vi "AlliGator Read HDF5 FLI Dataset Series Timestamps.vi"(8 "error in (no error)":errorcluster, 11 "File Paths":path[](array[path])) -> (0 "error out":errorcluster, 2 "Timestamps":dbl[](array[numeric]), 3 "File Paths (dup)":path[](array[path]))   [LabVIEW 2021, in "AlliGator HDF5.lvlib"]
doc: "Loads HDF5 FLI dataset gate images timestamps"
uses:
  AlliGator HDF5.lvlib
  <vilib>/addons/h5labview2/base/lib_path.vi
  <vilib>/addons/h5labview2/base/H5Equery.vi
  <vilib>/addons/h5labview2/base/hid_t.ctl
  <vilib>/addons/h5labview2/dataset/H5Dread.llb/H5Dread.xnode
  <vilib>/addons/h5labview2/file/H5F.lvlib
  <vilib>/addons/h5labview2/group/H5G.lvlib
  Error/Error.lvlib
panel:
  # "see the AlliGator License on the block diagram (Ctrl+E or Window:Show Block Diagram)"
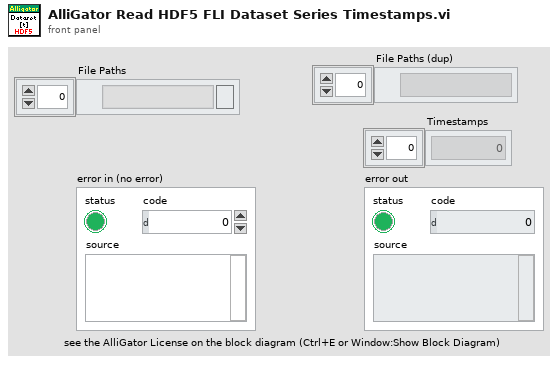
[diagram p1: front panel]
types:
  T1 = typedef "hid_t.ctl" = i64
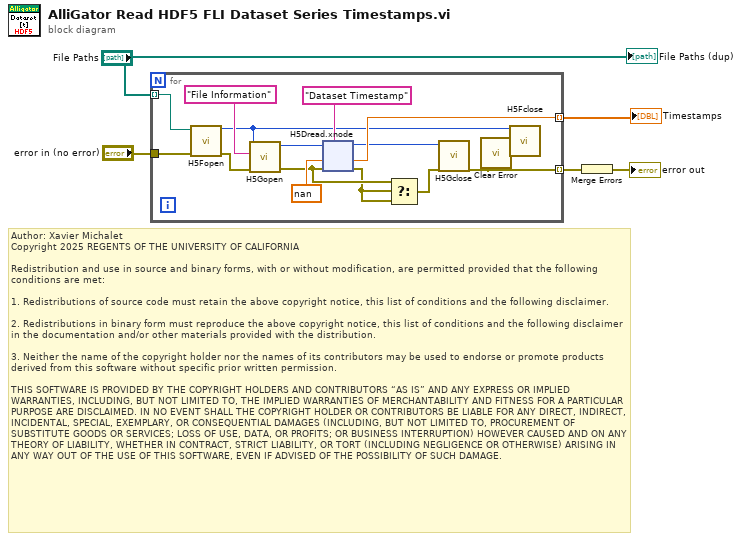
[diagram p0: block diagram]
diagram:
  # "Author: Xavier Michalet\nCopyright 2025 REGENTS OF THE UNIVERSITY OF CALIFORNIA\n\nRedistribution and use in source and binary forms, with or without modification, are permitted provided that the following conditions are met:\n\n1. Redistributions of source code must retain the above copyright notice, this list of conditions and the following disclaimer.\n\n2. Redistributions in binary form must reproduce the above copyright notice, this list of conditions and the following disclaimer in the documentation and/or other materials provided with the distribution.\n\n3. Neither the name of the copyright holder nor the names of its contributors may be used to endorse or promote products derived from this software without specific prior written permission.\n\nTHIS SOFTWARE IS PROVIDED BY THE COPYRIGHT HOLDERS AND CONTRIBUTORS “AS IS” AND ANY EXPRESS OR IMPLIED WARRANTIES, INCLUDING, BUT NOT LIMITED TO, THE IMPLIED WARRANTIES OF MERCHANTABILITY AND FITNESS FOR A PARTICULAR PURPOSE ARE DISCLAIMED. IN NO EVENT SHALL THE COPYRIGHT HOLDER OR CONTRIBUTORS BE LIABLE FOR ANY DIRECT, INDIRECT, INCIDENTAL, SPECIAL, EXEMPLARY, OR CONSEQUENTIAL DAMAGES (INCLUDING, BUT NOT LIMITED TO, PROCUREMENT OF SUBSTITUTE GOODS OR SERVICES; LOSS OF USE, DATA, OR PROFITS; OR BUSINESS INTERRUPTION) HOWEVER CAUSED AND ON ANY THEORY OF LIABILITY, WHETHER IN CONTRACT, STRICT LIABILITY, OR TORT (INCLUDING NEGLIGENCE OR OTHERWISE) ARISING IN ANY WAY OUT OF THE USE OF THIS SOFTWARE, EVEN IF ADVISED OF THE POSSIBILITY OF SUCH DAMAGE."
  n1 = for {
    tunnel: "File Paths" -> [w20] mode=indexing
    tunnel: "error in (no error)" -> [w19]
    tunnel: [w13] -> w3 mode=indexing
    tunnel: [w10] -> w2 mode=indexing
    n2 = call <vilib>:"H5Fopen.vi"("error in (no error)"=w19, "path"=w20) -> ("error out"=w17:errorcluster, "ref out"=w11:T1)  [unwired: 8 in]
    n3 = call <vilib>:"H5Gopen.vi"("error in (no error)"=w17, "name"="File Information", "ref in"=w11) -> ("error out"=w8:errorcluster, "group out"=w16:T1)  [unwired: 7 in]
    n4 = xnode "H5Dread.xnode"("dataset name (this)"="Dataset Timestamp" ("name"), "error in (no error)"=w8, "default"=nan ("Time Stamp Control"), "ref in"=w16) -> ("error out"=w7:errorcluster, "data"=w13:dbl, "ref out"=w12:T1)  [unwired: 2 in, 1 out]
    n5 = Select(t=w8, s=w7, f=w7) -> (s? t:f=w6:errorcluster)
    n6 = call <vilib>:"H5Gclose.vi"("error in (no error)"=w6, "group in"=w12) -> ("error out"=w10:errorcluster)  [unwired: 9 in]
    n7 = call "Clear Error.vi"("Error In"=w10) -> ("no Error Out"=w9:errorcluster)  [unwired: 8 in]
    n8 = call <vilib>:"H5Fclose.vi"("error in (no error)"=w9, "ref"=w11) -> ()  [unwired: 9 in, 1 out]
  }
  "Timestamps" <- w3
  n9 = Merge Errors(w2) -> (→"error out":errorcluster)
  "File Paths (dup)" <- "File Paths"
